vi "Init.vi"(7 "Name":string, 8 "error in (no error)":errorcluster, 10 "MSS":refnum<class "Measure and Stimulus Subsystems.lvclass">, 11 "Task Base in":refnum<class "Task Base.lvclass">) -> (0 "error out":errorcluster, 3 "Task Base out":refnum<class "Task Base.lvclass">)   [LabVIEW 2023, in "HAL GOOP4.lvlib" / "Task Base.lvclass"]
uses:
  Task Base.lvclass
  Measure and Stimulus Subsystems/Measure and Stimulus Subsystems.lvclass
  Task Base.lvclass/Task Base.ctl
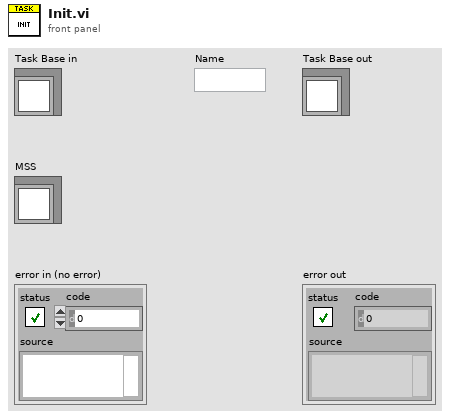
[diagram p1: front panel]
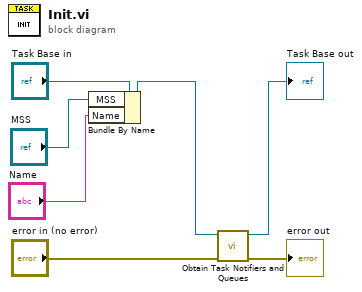
[diagram p0: block diagram]
diagram:
  n1 = Bundle By Name(cluster="Task Base in", "MSS"="MSS", "Name"="Name") -> (w3:refnum<class "Task Base.lvclass">)
  n2 = call-dynamic "Obtain Task Notifiers and Queues.vi"("error in (no error)"="error in (no error)", "Task Base in"=w3) -> ("error out"=→"error out":errorcluster, "Task Base out"=→"Task Base out":refnum<class "Task Base.lvclass">)  [unwired: 8 in]
